vi "Teleop.vi"(10 "Match Info":T1={"Autonomous Elapsed Seconds"=0.0, "TeleOp Elapsed Seconds"=0.0, "Disabled Elapsed Seconds"=0.0, "Visited Autonomous"=FALSE, "Visited TeleOp"=FALSE, "Visited Disabled"=FALSE, "Autonomous Settings"={"Autonomous Style"=enum."Independent", "VI Refnum"=refnum}}, 11 "Call Context":T2) -> ()   [LabVIEW 2012]
doc: "This VI is called for each TeleOp packet received from the DS where the robot is not disabled. It is often used to read from the joysticks and update I/O or to update setpoints for timed control loops. It should complete and return within 20 milliseconds or it may miss DS packets."
uses:
  <vilib>/Rock Robotics/WPI/DriverStation/WPI_DriverStationDerivedRobotMode.ctl
  <vilib>/Rock Robotics/WPI/DriverStation/WPI_DriverStationMatch Info.ctl
  Robot Global Data.vi
  <vilib>/Rock Robotics/WPI/Joystick/WPI_JoystickGetSetRefNum.vi
  <vilib>/Rock Robotics/WPI/RobotDrive/WPI_RobotDriveGetSetRefNum.vi
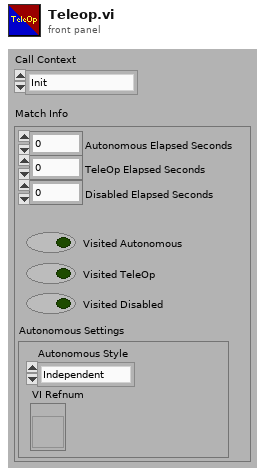
[diagram p1: front panel]
types:
  T1 = typedef "WPI_DriverStationMatch Info.ctl" = cluster{"Autonomous Elapsed Seconds":dbl, "TeleOp Elapsed Seconds":dbl, "Disabled Elapsed Seconds":dbl, "Visited Autonomous":bool, "Visited TeleOp":bool, "Visited Disabled":bool, "Autonomous Settings":cluster{"Autonomous Style":enum16{"Iterative", "Independent"}, "VI Refnum":refnum<vi>}}
  T2 = typedef "WPI_DriverStationDerivedRobotMode.ctl" = enum16{"Init", "Execute", "Stop"}
  T3 = typedef "WPI_JoystickDevRef.ctl" = cluster{"Device":T4}
  T4 = typedef "WPI_JoystickDeviceEnum.ctl" = enum16{"USB 1", "USB 2", "USB 3", "USB 4", "Kinect 1", "Kinect 2"}
  T5 = typedef "WPI_JoystickButtonState.ctl" = cluster{"Button 1":bool, "Button 2":bool, "Button 3":bool, "Button 4":bool, "Button 5":bool, "Button 6":bool, "Button 7":bool, "Button 8":bool, "Button 9":bool, "Button 10":bool, "Button 11":bool, "Button 12":bool}
  T6 = cluster{"axis 1 (x)":dbl, "axis 2 (y)":dbl, "axis 3 (throttle)":dbl, "axis 4":dbl, "axis 5":dbl, "axis 6":dbl}
  T7 = typedef "WPI_RobotDriveDevRef.ctl" = cluster{"DevStatus":errorcluster, "Motors[]":T8[], "Square Inputs":bool, "Max Output":dbl, "Isochronous":bool}
  T8 = typedef "WPI_MotorControlDeviceRef.ctl" = cluster{"DeviceStatus":errorcluster, "Type":enum16{"PWM", "CAN"}, "PWM":cluster{"Digital Module":T9, "PWM Channel":T10, "DeadBand":T11}, "CAN":cluster{"Device Number":u8, "Control Mode":T12, "Semaphore":T13, "Max Vout":dbl}, "Invert":bool, "TransformRef":T14, "InvTransformRef":T14}
  T9 = typedef "FPGA_TypedefDigitalModule.ctl" = enum16{"Digital Module 1", "Digital Module 2"}
  T10 = typedef "FPGA_DIOPWMChannel.ctl" = enum8{"PWM 1", "PWM 2", "PWM 3", "PWM 4", "PWM 5", "PWM 6", "PWM 7", "PWM 8", "PWM 9", "PWM 10", "Invalid"}
  T11 = typedef "WPI_PWMDeadband.ctl" = cluster{"Name":string, "maxPositivePwm":i32, "minPositivePwm":i32, "centerPwm":i32, "maxNegativePwm":i32, "minNegativePwm":i32, "angularRange":u16}
  T12 = typedef "WPI_CANJaguar_ControlMode.ctl" = enum8{"Percent VBus", "Current", "Speed", "Position", "Voltage"}
  T13 = typedef "Semaphore RefNum" = refnum<k1>
  T14 = typedef "WPI_PWMTransform_ConPane.ctl" = refnum<vi>
  T15 = cluster{"Shoot":bool, "Enable_Targeting":bool, "Shooter":dbl, "LeadScrew":dbl, "Feed":bool, "Pickup":bool}
  T16 = cluster{"PizzaLow":dbl, "PizzaMid":dbl, "PizzaTop":dbl}
  T17 = typedef "WPI_DigitalInputDevRef.ctl" = cluster{"DevStatus":errorcluster, "DIO Channel":T18, "Digital Module":T9}
  T18 = typedef "FPGA_DIOChannel.ctl" = enum8{"DIO 1", "DIO 2", "DIO 3", "DIO 4", "DIO 5", "DIO 6", "DIO 7", "DIO 8", "DIO 9", "DIO 10", "DIO 11", "DIO 12", "DIO 13", "DIO 14", "Invalid"}
  T19 = cluster{"Frisbee_Catch":bool, "Shooter_Ready":bool, "LeadScrewEnd":bool}
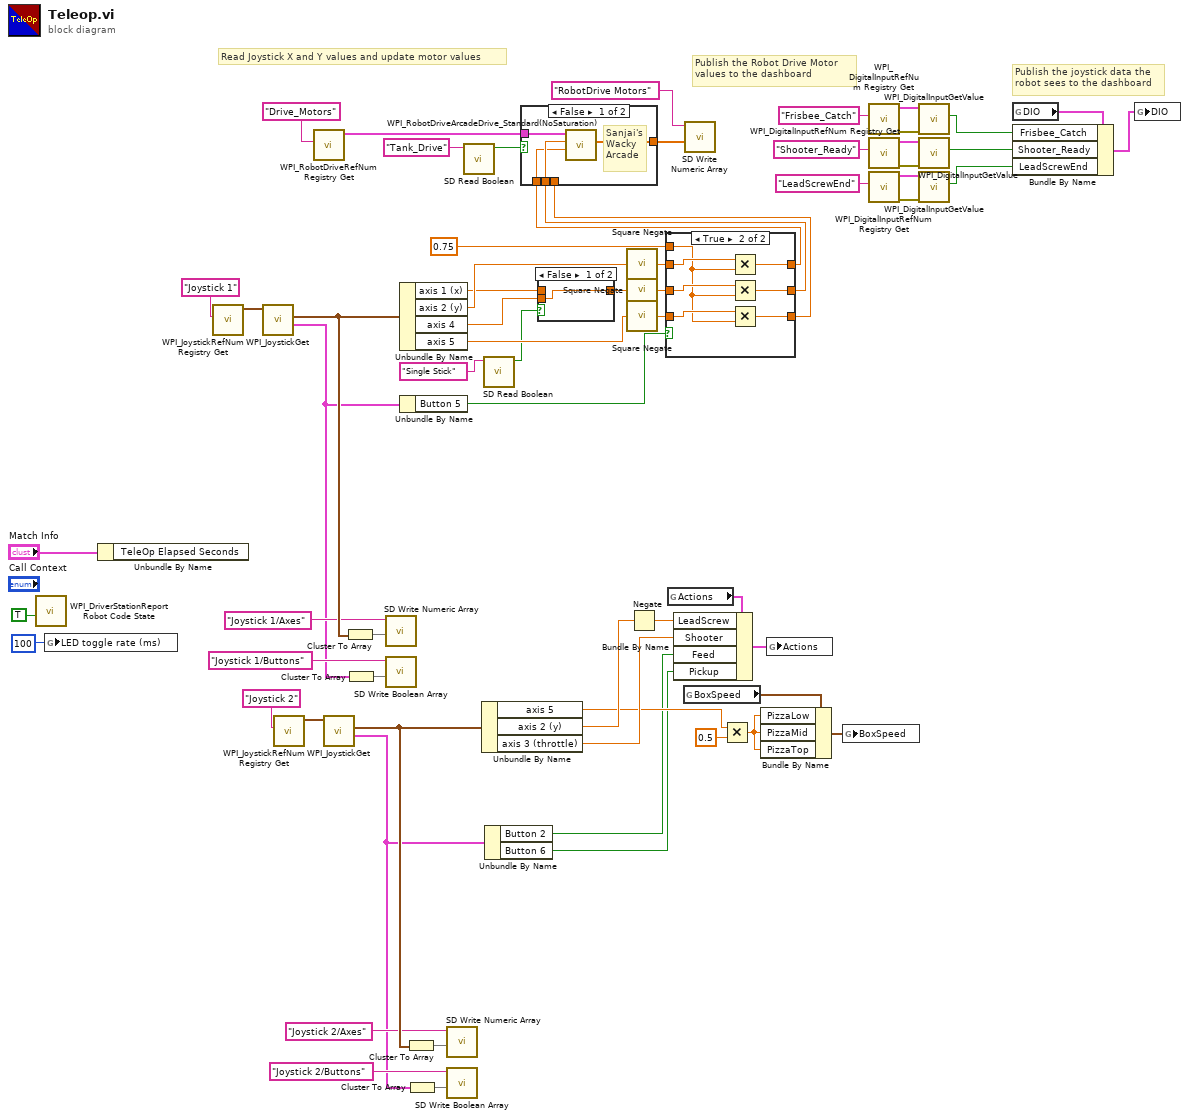
[diagram p0: block diagram]
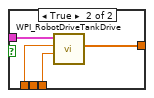
[diagram p4: hidden frame]
diagram:
  # "Publish the Robot Drive Motor\nvalues to the dashboard"
  # "Publish the joystick data the\nrobot sees to the dashboard"
  # "Read Joystick X and Y values and update motor values"
  n1 = call <vilib>:"WPI_DriverStationReport Robot Code State.vi"("TeleOp"=TRUE ("Autonomous")) -> ()  [unwired: 10 in, 1 out]
  n2 = global write "Robot Global Data.vi" "LED toggle rate (ms)"(u32 100 ("LED ms toggle rate")) -> ()
  n3 = Unbundle By Name("Match Info") -> ()  [unwired: 1 out]
  n4 = call <vilib>:"WPI_JoystickRefNum Registry Get.vi"("refnum name"="Joystick 1") -> ("JoystickDevRef"=w61:T3)  [unwired: 1 in, 9 out]
  n5 = call <vilib>:"WPI_JoystickGet.vi"("JoystickDevRef"=w61) -> ("Buttons"=w51:T5, "Axes"=w58:T6)  [unwired: 1 in, 4 out]
  n6 = call <vilib>:"WPI_JoystickRefNum Registry Get.vi"("refnum name"="Joystick 2") -> ("JoystickDevRef"=w40:T3)  [unwired: 1 in, 9 out]
  n7 = call <vilib>:"WPI_RobotDriveRefNum Registry Get.vi"("refnum name"="Drive_Motors") -> ("RobotDriveDevRef"=w63:T7)  [unwired: 1 in, 9 out]
  n8 = call <vilib>:"WPI_JoystickGet.vi"("JoystickDevRef"=w40) -> ("Buttons"=w34:T5, "Axes"=w37:T6)  [unwired: 1 in, 4 out]
  n9 = Cluster To Array(cluster=w58) -> (array=w57:dbl[])
  n10 = Cluster To Array(cluster=w51) -> (array=w60:bool[])
  n11 = call <vilib>:"SD Write Numeric Array.vi"("Numeric Array"=w57, "Name"="Joystick 1/Axes") -> ()  [unwired: 8 in, 2 out]
  n12 = call <vilib>:"SD Write Boolean Array.vi"("Boolean Array"=w60, "Name"="Joystick 1/Buttons") -> ()  [unwired: 8 in, 2 out]
  n13 = Unbundle By Name(w58) -> ("axis 1 (x)"=w5:dbl, "axis 2 (y)"=w13:dbl, "axis 4"=w4:dbl, "axis 5"=w8:dbl)
  n14 = Unbundle By Name(w51) -> ("Button 5"=w31:bool)
  n15 = Cluster To Array(cluster=w37) -> (array=w36:dbl[])
  n16 = Cluster To Array(cluster=w34) -> (array=w39:bool[])
  n17 = call <vilib>:"SD Write Numeric Array.vi"("Numeric Array"=w36, "Name"="Joystick 2/Axes") -> ()  [unwired: 8 in, 2 out]
  n18 = call <vilib>:"SD Write Boolean Array.vi"("Boolean Array"=w39, "Name"="Joystick 2/Buttons") -> ()  [unwired: 8 in, 2 out]
  n19 = call <vilib>:"SD Read Boolean.vi"("Name"="Tank_Drive") -> ("Boolean"=w53:bool)  [unwired: 8 in, 2 out]
  n20 = Unbundle By Name(w37) -> ("axis 5"=w16:dbl, "axis 2 (y)"=w23:dbl, "axis 3 (throttle)"=w24:dbl)
  n21 = call <vilib>:"SD Read Boolean.vi"("Name"="Single Stick") -> ("Boolean"=w2:bool)  [unwired: 8 in, 2 out]
  n22 = Unbundle By Name(w34) -> ("Button 2"=w7:bool, "Button 6"=w6:bool)
  n23 = case shown="False" w2 {
    tunnel: w5 -> [_ w68]
    tunnel: w4 -> [w67 _]
    tunnel: [w67 w68] -> w3
    frame False {
    }
    frame True {
    }
  }
  n24 = call "Square Negate.vi"("x"=w13) -> ("x脖"=w14:dbl)
  n25 = call "Square Negate.vi"("x"=w3) -> ("x脖"=w12:dbl)
  n26 = call "Square Negate.vi"("x"=w8) -> ("x脖"=w15:dbl)
  n27 = Negate(x=w23) -> (-x=w22:dbl)
  n28 = case shown="True" w31 {
    tunnel: w14 -> [w69 w78]
    tunnel: w15 -> [w70 w77]
    tunnel: w12 -> [w71 w76]
    tunnel: [w71 w73] -> w10
    tunnel: [w69 w75] -> w11
    tunnel: [w70 w74] -> w9
    tunnel: 0.75 -> [_ w72]
    frame False {
    }
    frame True {
      n29 = Multiply(x=w78, y=w72) -> (x*y=w75:dbl)
      n30 = Multiply(x=w76, y=w72) -> (x*y=w73:dbl)
      n31 = Multiply(x=w77, y=w72) -> (x*y=w74:dbl)
    }
  }
  n32 = case shown="False" w53 {
    tunnel: w63 -> [w82 w85]
    tunnel: [w81 w86] -> w54
    tunnel: w9 -> [_ w84]
    tunnel: w10 -> [w80 _]
    tunnel: w11 -> [w79 w83]
    frame False {
      # "Sanjai's\nWacky\nArcade"
      n33 = call <vilib>:"WPI_RobotDriveArcadeDrive_Standard(NoSaturation).vi"("Y axis value"=w79, "X axis value"=w80, "RobotDriveDevRef"=w82) -> ("Motor Values"=w81:dbl[])  [unwired: 1 in, 7 out]
    }
    frame True {
      n34 = call <vilib>:"WPI_RobotDriveTankDrive.vi"("Right axis value"=w84, "Left axis value"=w83, "RobotDriveDevRef"=w85) -> ("Motor Values"=w86:dbl[])  [unwired: 6 in, 2 out]
    }
  }
  n35 = global read "Robot Global Data.vi" "Actions"() -> (w26:T15)
  n36 = Bundle By Name(cluster=w26, "LeadScrew"=w22, "Shooter"=w24, "Feed"=w7, "Pickup"=w6) -> (w25:T15)
  n37 = global read "Robot Global Data.vi" "BoxSpeed"() -> (w21:T16)
  n38 = call <vilib>:"SD Write Numeric Array.vi"("Numeric Array"=w54, "Name"="RobotDrive Motors") -> ()  [unwired: 8 in, 2 out]
  n39 = Multiply(x=w16, y=0.5) -> (x*y=w19:dbl)
  n40 = Bundle By Name(cluster=w21, "PizzaLow"=w19, "PizzaMid"=w19, "PizzaTop"=w19) -> (w20:T16)
  n41 = global write "Robot Global Data.vi" "Actions"(w25) -> ()
  n42 = global write "Robot Global Data.vi" "BoxSpeed"(w20) -> ()
  n43 = call <vilib>:"WPI_DigitalInputRefNum Registry Get.vi"("refnum name"="Frisbee_Catch") -> ("error out"=w42:errorcluster, "DigitalInputDevRef"=w43:T17)  [unwired: 9 in]
  n44 = call <vilib>:"WPI_DigitalInputRefNum Registry Get.vi"("refnum name"="Shooter_Ready") -> ("error out"=w45:errorcluster, "DigitalInputDevRef"=w44:T17)  [unwired: 9 in]
  n45 = call <vilib>:"WPI_DigitalInputRefNum Registry Get.vi"("refnum name"="LeadScrewEnd") -> ("error out"=w29:errorcluster, "DigitalInputDevRef"=w28:T17)  [unwired: 9 in]
  n46 = call <vilib>:"WPI_DigitalInputGetValue.vi"("error in (no error)"=w42, "DigitalInputDevRef"=w43) -> ("Value"=w18:bool)  [unwired: 7 in, 2 out]
  n47 = call <vilib>:"WPI_DigitalInputGetValue.vi"("error in (no error)"=w45, "DigitalInputDevRef"=w44) -> ("Value"=w41:bool)  [unwired: 7 in, 2 out]
  n48 = call <vilib>:"WPI_DigitalInputGetValue.vi"("error in (no error)"=w29, "DigitalInputDevRef"=w28) -> ("Value"=w27:bool)  [unwired: 7 in, 2 out]
  n49 = global read "Robot Global Data.vi" "DIO"() -> (w49:T19)
  n50 = Bundle By Name(cluster=w49, "Frisbee_Catch"=w18, "Shooter_Ready"=w41, "LeadScrewEnd"=w27) -> (w48:T19)
  n51 = global write "Robot Global Data.vi" "DIO"(w48) -> ()
